vi "Symphony GetProgPar.vi"(0 "Param":enum16{"InitVal", "Tous"}(ring)=enum."Tous", 11 "error in":errorcluster) -> (1 "Y Bins":i32=1 min=1 max=256 step=1, 2 "X Start":i32=1 min=1 max=1024 step=1, 3 "X End":i32=1024 min=1 max=1024 step=1, 4 "ImageMode":bool, 6 "Shutter Enable":bool=TRUE, 8 "InitOnStart":bool=TRUE, 10 "Launch server":bool=TRUE, 12 "ADC":u16, 13 "Gain":u16=2, 14 "Int_time(ms)":i16=10 caption="Integration time(ms)", 15 "error out":errorcluster)   [LabVIEW 2012]
doc: "Ce Vi enregistre les paramètres des différents axes dans un fichier .ini"
uses:
  <vilib>/Utility/config.llb/Read Key (Boolean).vi
  <vilib>/Utility/config.llb/Read Key (I32).vi
  <vilib>/Utility/config.llb/NI_LVConfig.lvlib
panel:
  out "Accumulations:":u16=1 caption="Accumulations" min=1 step=1
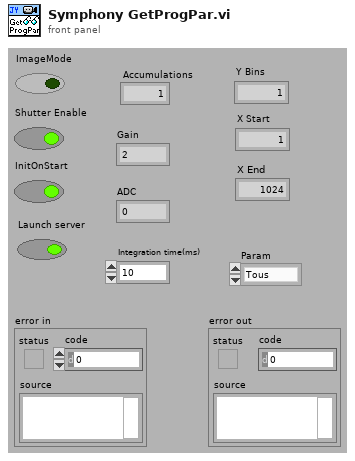
[diagram p1: front panel]
types:
  T1 = typedef "NI_LVConfig.lvlib/Config Data RefNum.ctl" = refnum<k1>
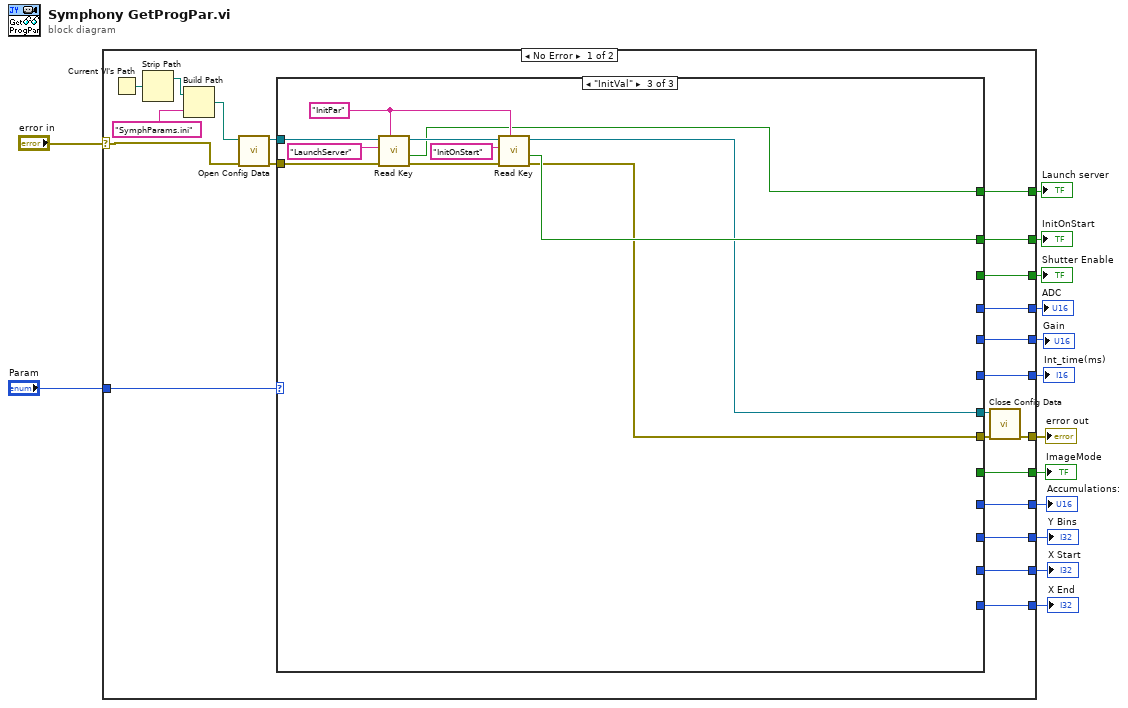
[diagram p0: block diagram]
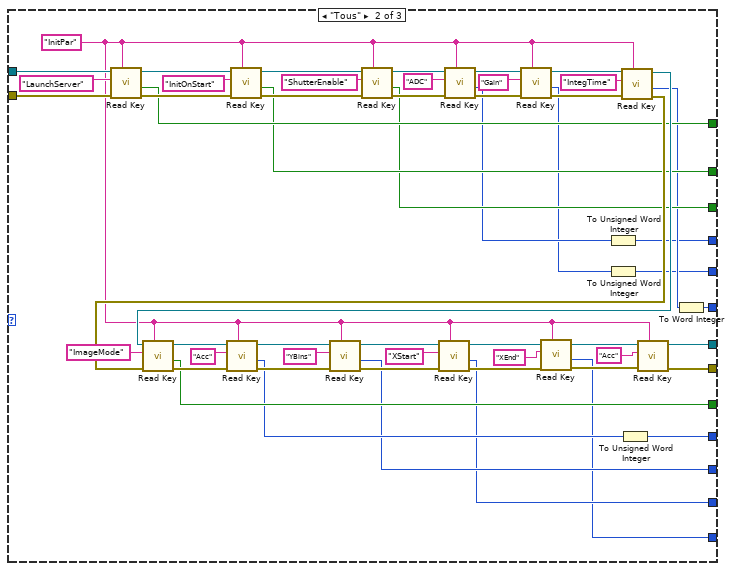
[diagram p3: hidden frame]
diagram:
  n1 = case shown="No Error" "error in" {
    selector: "error in" -> [w27 w104]
    tunnel: [w31 w104] -> w14
    tunnel: [w26 _] -> w12
    tunnel: [w25 _] -> w11
    tunnel: [w24 _] -> w10
    tunnel: [w23 _] -> w9
    tunnel: [w22 _] -> w8
    tunnel: [w21 _] -> w7
    tunnel: [w20 _] -> w6
    tunnel: [w19 _] -> w5
    tunnel: [w18 _] -> w4
    tunnel: [w17 _] -> w3
    tunnel: [w16 _] -> w2
    tunnel: "Param" -> [w15 _]
    frame No Error {
      n2 = Current VI's Path() -> (path=w36:path)
      n3 = Strip Path(path=w36) -> (stripped path=w28:path)  [unwired: 1 out]
      n4 = Build Path(base path=w28, name or relative path="SymphParams.ini") -> (appended path=w34:path)
      n5 = call <vilib>:"Open Config Data.vi"("error in (no error)"=w27, "configuration file path"=w34) -> ("error out"=w32:errorcluster, "refnum"=w33:T1)  [unwired: 7 in, 1 out]
      n6 = case shown="\"InitVal\"" w15 {
        tunnel: w33 -> [w38 w84 w102]
        tunnel: w32 -> [w37 w83 w101]
        tunnel: [w37 w56 w94] -> w30
        tunnel: [w38 w55 w95] -> w29
        tunnel: [_ w53 w93] -> w26
        tunnel: [_ w52 w96] -> w25
        tunnel: [_ w51 _] -> w24
        tunnel: [_ w47 _] -> w23
        tunnel: [_ w46 _] -> w22
        tunnel: [_ w45 _] -> w21
        tunnel: [_ w44 _] -> w20
        tunnel: [_ w42 _] -> w19
        tunnel: [_ w41 _] -> w18
        tunnel: [_ w40 _] -> w17
        tunnel: [_ w39 _] -> w16
        frame Default {
          # "choix invalide!"
        }
        frame "Tous" {
          w54 = "InitPar" ("section")
          n7 = call-poly <vilib>:"Read Key.vi"("section"=w54, "error in (no error)"=w83, "key"="LaunchServer", "refnum"=w84) -> ("error out"=w80:errorcluster, "value"=w53:bool, "refnum out"=w82:T1)  [unwired: 4 in, 1 out]
          n8 = call-poly <vilib>:"Read Key.vi"("section"=w54, "error in (no error)"=w80, "key"="InitOnStart", "refnum"=w82) -> ("error out"=w79:errorcluster, "value"=w52:bool, "refnum out"=w74:T1)  [unwired: 4 in, 1 out]
          n9 = call-poly <vilib>:"Read Key.vi"("section"=w54, "error in (no error)"=w79, "key"="ShutterEnable", "refnum"=w74) -> ("error out"=w78:errorcluster, "value"=w51:bool, "refnum out"=w75:T1)  [unwired: 4 in, 1 out]
          n10 = call-poly <vilib>:"Read Key.vi"("section"=w54, "error in (no error)"=w78, "key"="ADC", "refnum"=w75) -> ("error out"=w77:errorcluster, "value"=w50:i32, "refnum out"=w76:T1)  [unwired: 4 in, 1 out]
          n11 = call-poly <vilib>:"Read Key.vi"("section"=w54, "error in (no error)"=w77, "key"="Gain", "refnum"=w76) -> ("error out"=w61:errorcluster, "value"=w49:i32, "refnum out"=w60:T1)  [unwired: 4 in, 1 out]
          n12 = To Unsigned Word Integer(number=w50) -> (unsigned 16bit integer=w47:u16)
          n13 = To Unsigned Word Integer(number=w49) -> (unsigned 16bit integer=w45:u16)
          n14 = call-poly <vilib>:"Read Key.vi"("section"=w54, "error in (no error)"=w61, "key"="IntegTime", "refnum"=w60) -> ("error out"=w63:errorcluster, "value"=w48:i32, "refnum out"=w62:T1)  [unwired: 4 in, 1 out]
          n15 = call-poly <vilib>:"Read Key.vi"("section"=w54, "error in (no error)"=w63, "key"="ImageMode", "refnum"=w62) -> ("error out"=w72:errorcluster, "value"=w44:bool, "refnum out"=w73:T1)  [unwired: 4 in, 1 out]
          n16 = call-poly <vilib>:"Read Key.vi"("section"=w54, "error in (no error)"=w72, "key"="Acc", "refnum"=w73) -> ("error out"=w70:errorcluster, "value"=w43:i32, "refnum out"=w71:T1)  [unwired: 4 in, 1 out]
          n17 = call-poly <vilib>:"Read Key.vi"("section"=w54, "error in (no error)"=w70, "key"="YBins", "refnum"=w71) -> ("error out"=w68:errorcluster, "value"=w41:i32, "refnum out"=w69:T1)  [unwired: 4 in, 1 out]
          n18 = call-poly <vilib>:"Read Key.vi"("section"=w54, "error in (no error)"=w68, "key"="XStart", "refnum"=w69) -> ("error out"=w67:errorcluster, "value"=w40:i32, "refnum out"=w66:T1)  [unwired: 4 in, 1 out]
          n19 = call-poly <vilib>:"Read Key.vi"("section"=w54, "error in (no error)"=w67, "key"="XEnd", "refnum"=w66) -> ("error out"=w57:errorcluster, "value"=w39:i32, "refnum out"=w58:T1)  [unwired: 4 in, 1 out]
          n20 = To Unsigned Word Integer(number=w43) -> (unsigned 16bit integer=w42:u16)
          n21 = call-poly <vilib>:"Read Key.vi"("section"=w54, "error in (no error)"=w57, "key"="Acc", "refnum"=w58) -> ("error out"=w56:errorcluster, "refnum out"=w55:T1)  [unwired: 4 in, 2 out]
          n22 = To Word Integer(number=w48) -> (16bit integer=w46:i16)
        }
        frame "InitVal" {
          w97 = "InitPar" ("section")
          n23 = call-poly <vilib>:"Read Key.vi"("section"=w97, "error in (no error)"=w101, "key"="LaunchServer", "refnum"=w102) -> ("error out"=w98:errorcluster, "value"=w93:bool, "refnum out"=w100:T1)  [unwired: 4 in, 1 out]
          n24 = call-poly <vilib>:"Read Key.vi"("section"=w97, "error in (no error)"=w98, "key"="InitOnStart", "refnum"=w100) -> ("error out"=w94:errorcluster, "value"=w96:bool, "refnum out"=w95:T1)  [unwired: 4 in, 1 out]
        }
      }
      n25 = call <vilib>:"Close Config Data.vi"("error in (no error)"=w30, "refnum"=w29) -> ("error out"=w31:errorcluster)  [unwired: 8 in, 1 out]
    }
    frame Error {
    }
  }
  "error out" <- w14
  "Shutter Enable" <- w10
  "InitOnStart" <- w11
  "Launch server" <- w12
  "Int_time(ms)" <- w8
  "ADC" <- w9
  "Gain" <- w7
  "Accumulations:" <- w5
  "ImageMode" <- w6
  "Y Bins" <- w4
  "X Start" <- w3
  "X End" <- w2
